vi "listAllTestMethods.vi"(8 "error in (no error)":errorcluster, 11 "MyFirstTest in":refnum<class "MyFirstTest.lvclass">) -> (0 "error out":errorcluster, 2 "test methods":string[](array[string]), 3 "MyFirstTest out":refnum<class "MyFirstTest.lvclass">)   [LabVIEW 2011, in "MyFirstTest.lvclass"]
doc: "List all test methods that are members of the current TestCase class."
uses:
  MyFirstTest.lvclass
panel:
  # "JKI VI Tester for LabVIEW\nhttp://jkisoft.com/vi-tester\nCopyright (C) 2007-2009, JKI <info@jkisoft.com>\nALL RIGHTS RESERVED"
  # "Copyright © 2007 James Kring, Inc. All rights reserved.\n\nAuthor: Jim Kring [jim.kring@jameskring.com]\n\nThis library is provided \"AS IS\" ,WITHOUT WARRANTIES OR \nCONDITIONS OF ANY KIND, either express or implied.\n\nJames Kring, Inc. -- http://www.jameskring.com"
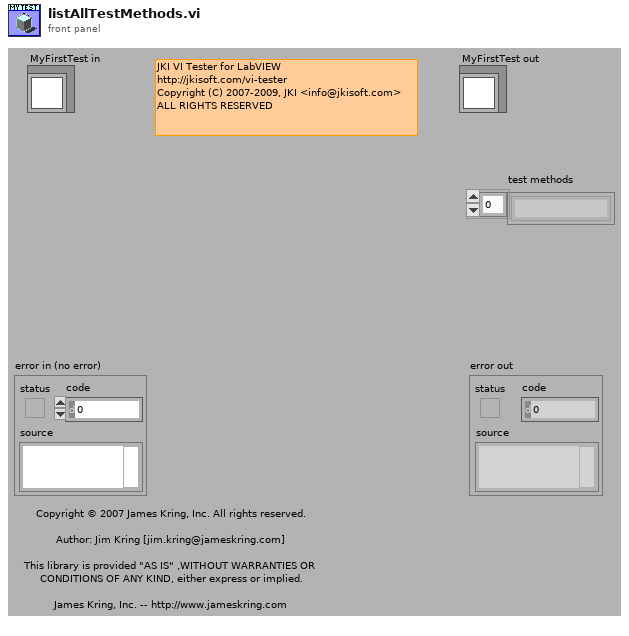
[diagram p1: front panel]
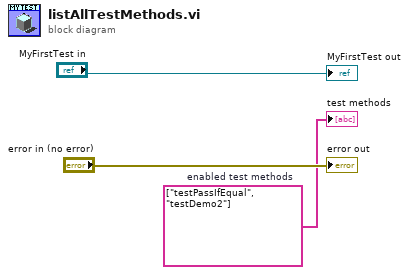
[diagram p0: block diagram]
diagram:
  w1 = string[] ["testPassIfEqual", "testDemo2"]  # enabled test methods
  "error out" <- "error in (no error)"
  "MyFirstTest out" <- "MyFirstTest in"
  "test methods" <- w1
